vi "Read Temperature.vi"(11 "error in (no error)":errorcluster) -> (6 "Air Temperature (°C)":dbl min=25.0 max=80.0 step=0.1, 15 "error out":errorcluster)   [LabVIEW 2010]
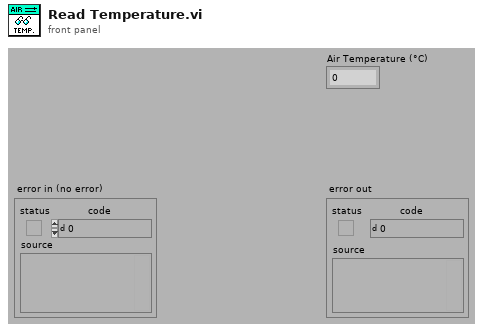
[diagram p1: front panel]
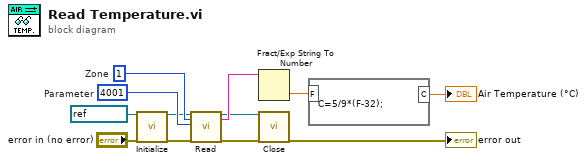
[diagram p0: block diagram]
diagram:
  w5 = u8 1  # Zone
  w6 = u32 4001  # Parameter
  n1 = call <instrlib>:"Initialize.vi"("Comms Port"=refnum<visa-resource-name> "COM3", "Error In"="error in (no error)") -> ("UUT Port 2"=w1:refnum<visa-resource-name>, "Error Out"=w8:errorcluster)  [unwired: 16 out]
  n2 = call <instrlib>:"Read.vi"("PC Comms Port"=w1, "Zone"=w5, "Parameter"=w6, "Error In"=w8) -> ("Read Value"=w2:string, "Error Out"=w7:errorcluster)  [unwired: 14 in]
  n3 = Fract/Exp String To Number(string=w2) -> (number=w4:dbl)  [unwired: 3 in, 1 out]
  n4 = call <instrlib>:"Close.vi"("PC Comms Port"=w1, "Error In"=w7) -> ("Error Out"=→"error out":errorcluster)  [unwired: 17 out]
  n5 = formula code="C=5/9*(F-32);"("F"=w4) -> ("C"=→"Air Temperature (°C)":dbl)
